vi "禹山浊度校准.vi"() -> ()   [LabVIEW 2016, in "斯坦道多参数.lvlib"]
uses:
  <vilib>/Utility/miscctls.llb/LVPointTypeDef.ctl
  <vilib>/Analysis/NI_AALBase.lvlib
  <vilib>/Analysis/NI_AALPro.lvlib
panel:
  out "滤波设定":dbl
  out "通讯状态":string
  out "第二点校准值":dbl
  out "第一点校准值":dbl
  out "最小值":sgl format="%.2g"
  out "最大值":sgl format="%.2g"
  in  "校准停止":bool
  in  "校准模式":u16(ring) items=["两点校准", "单点校准"]
  in  "标液2":dbl
  in  "标液1":dbl
  out "波形图表":sgl(graph) caption="历史曲线"
  out "温度测量值":dbl caption="温度" format="%#.2f"
  out "变异系数":dbl format="%.6g"
  out "standard deviation":dbl caption="标准差" format="%0.2f"
  out "mean":dbl caption="均值" format="%0.2f"
  out "提示":string
  in  "校准启动":bool
  out "测试值":dbl format="%#.2f"
  out "电极斜率":dbl format="%#.6f"
  out "电极零点":dbl format="%#.6f"
  # "浊度电极设定"
  # "℃"
  # "NTU"
  # "请选择校准模式:"
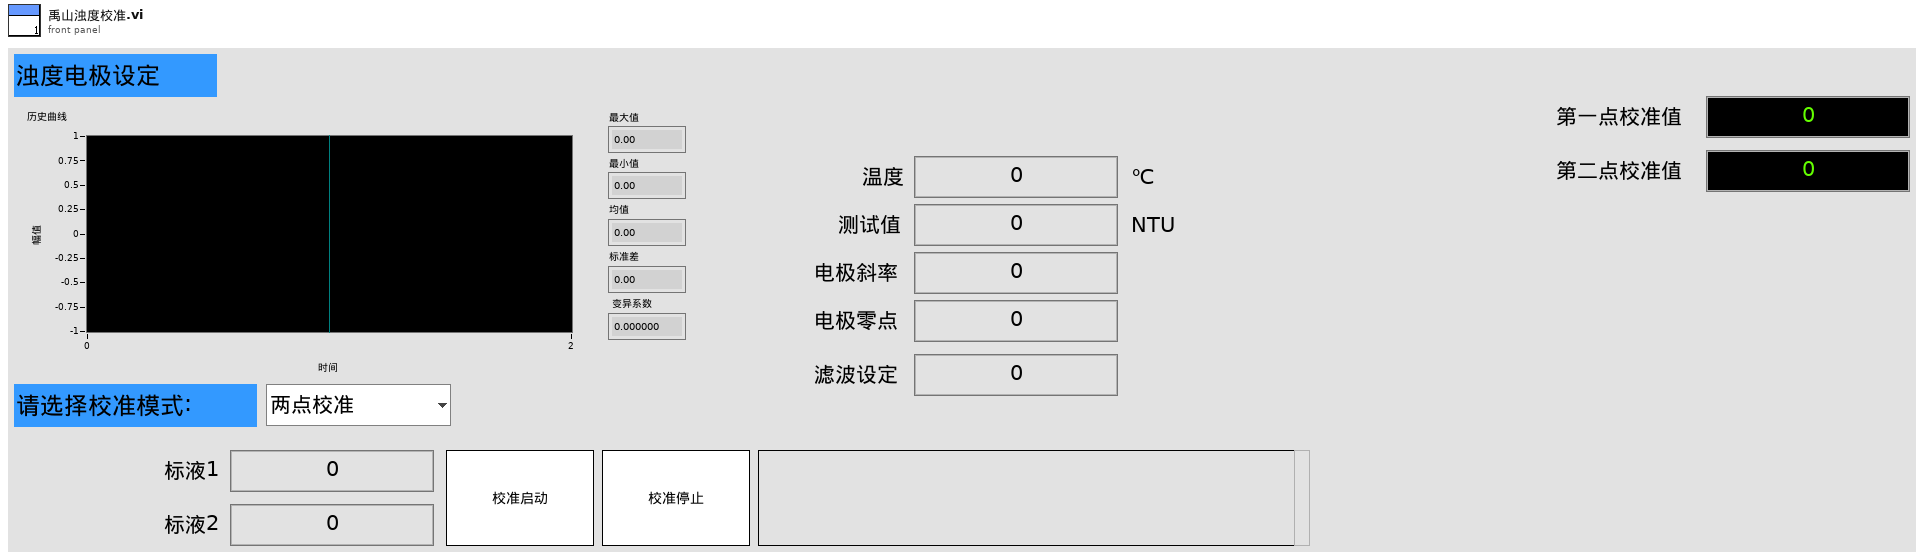
[diagram p1: front panel]
types:
  T1 = typedef "斯坦道多参数.lvlib/通知队列类型.ctl" = enum16{"pH", "DO", "DO2", "Cond", "Turb", "ORP", "叶绿素a", "藻密度", "COD"}
  T2 = typedef "LVPointTypeDef.ctl" = cluster{"Horizontal":i16, "Vertical":i16}
  T3 = cluster{"pH":u32, "DO":u32, "Cond":u32, "Turb":u32, "叶绿素a":u32, "藻密度":u32, "ORP":u32, "COD":u32}
  T4 = enum8{"Enabled", "Disabled", "Disabled and Grayed Out"}
  T5 = cluster{"ph":bool, "DO":bool, "Cond":bool, "Turb":bool, "叶绿素a":bool, "藻密度":bool, "ORP":bool, "COD":bool, "DO2":bool}
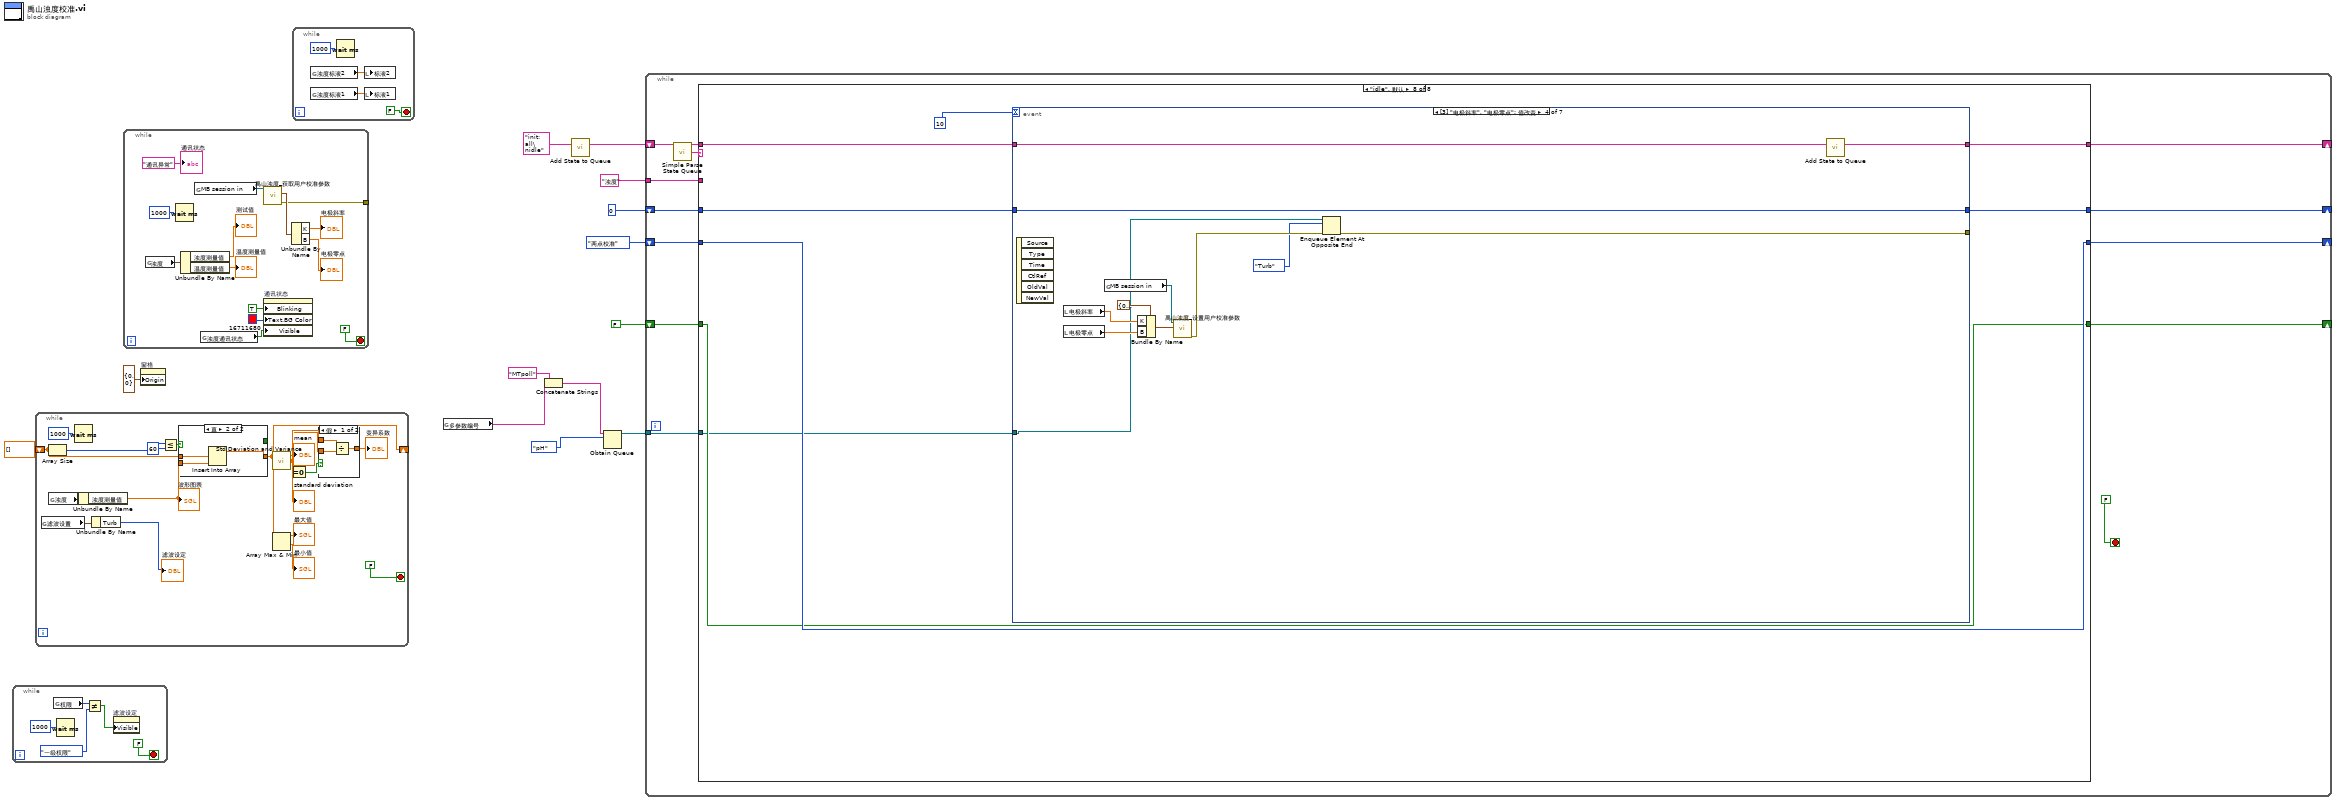
[diagram p0: block diagram]
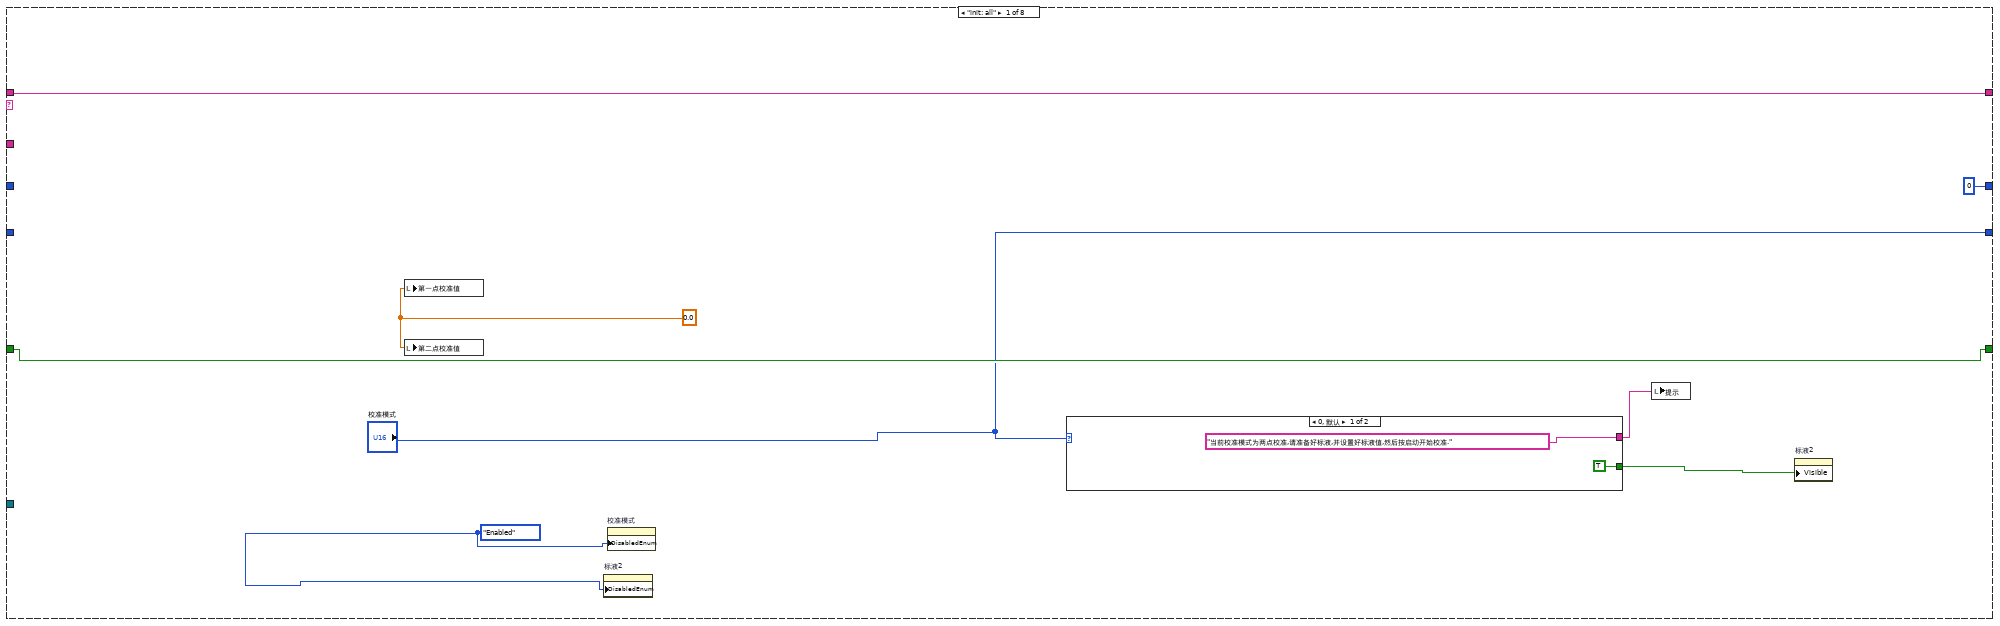
[diagram p2: hidden frame]
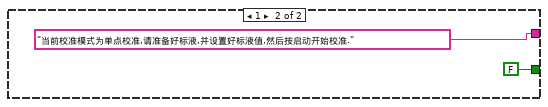
[diagram p3: hidden frame]
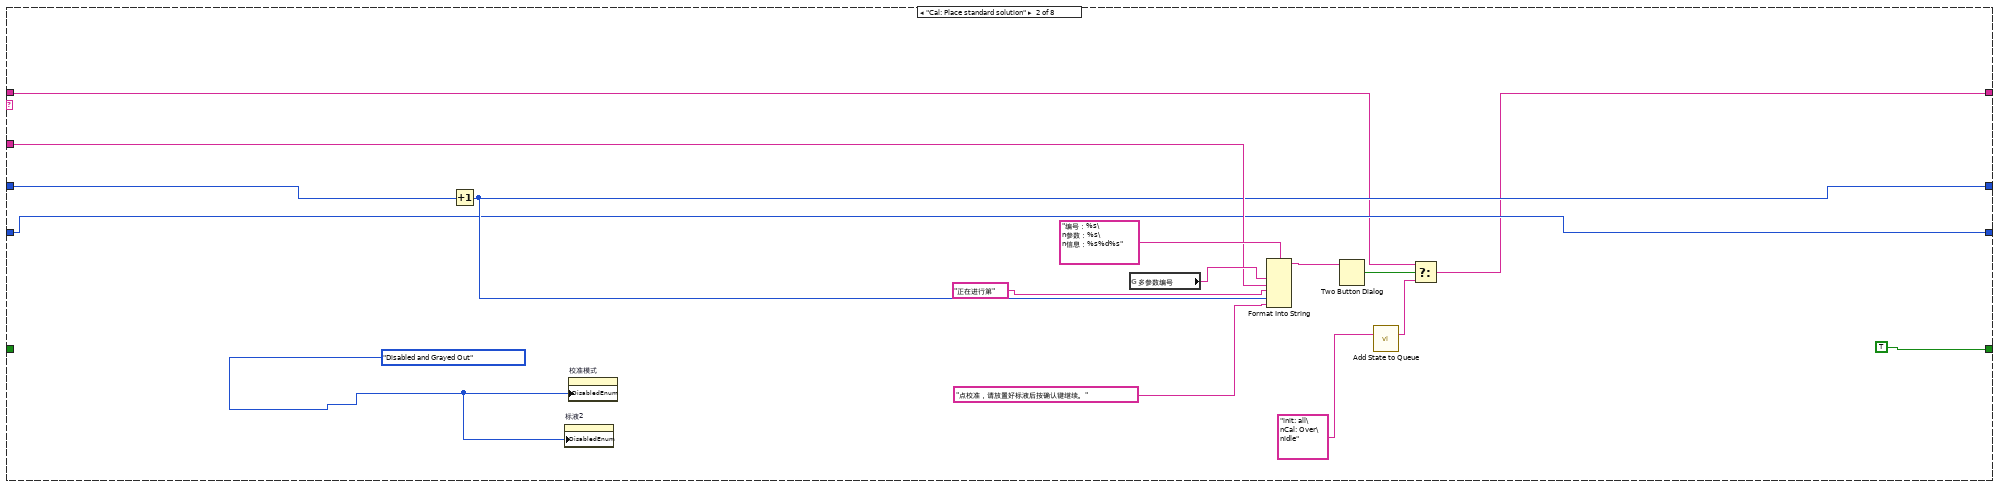
[diagram p4: hidden frame]
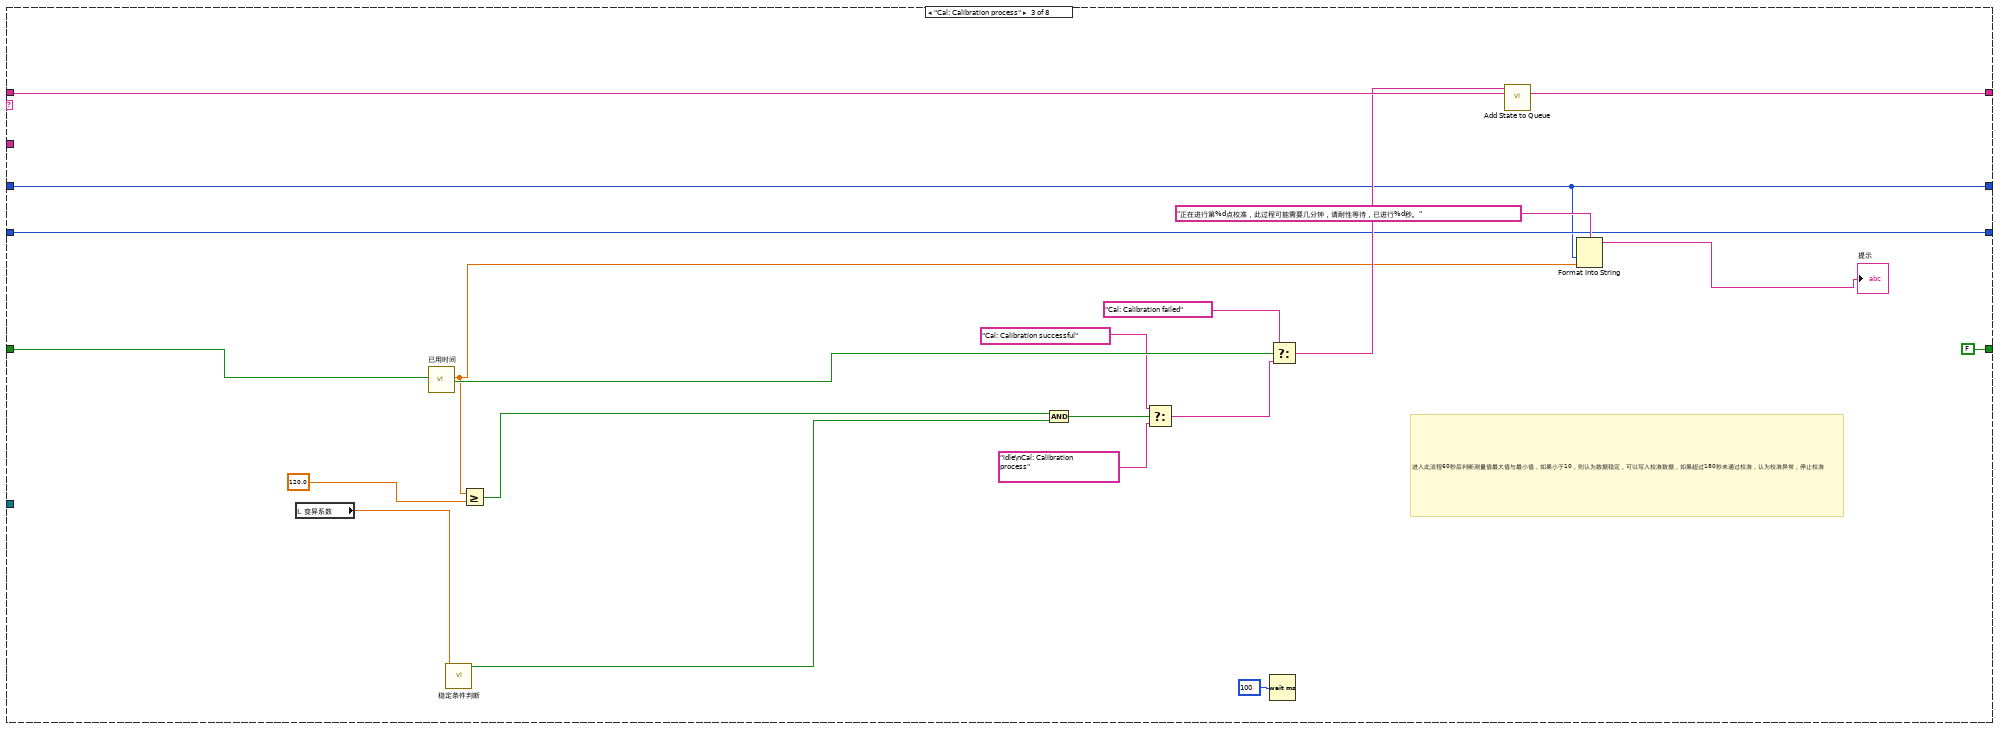
[diagram p5: hidden frame]
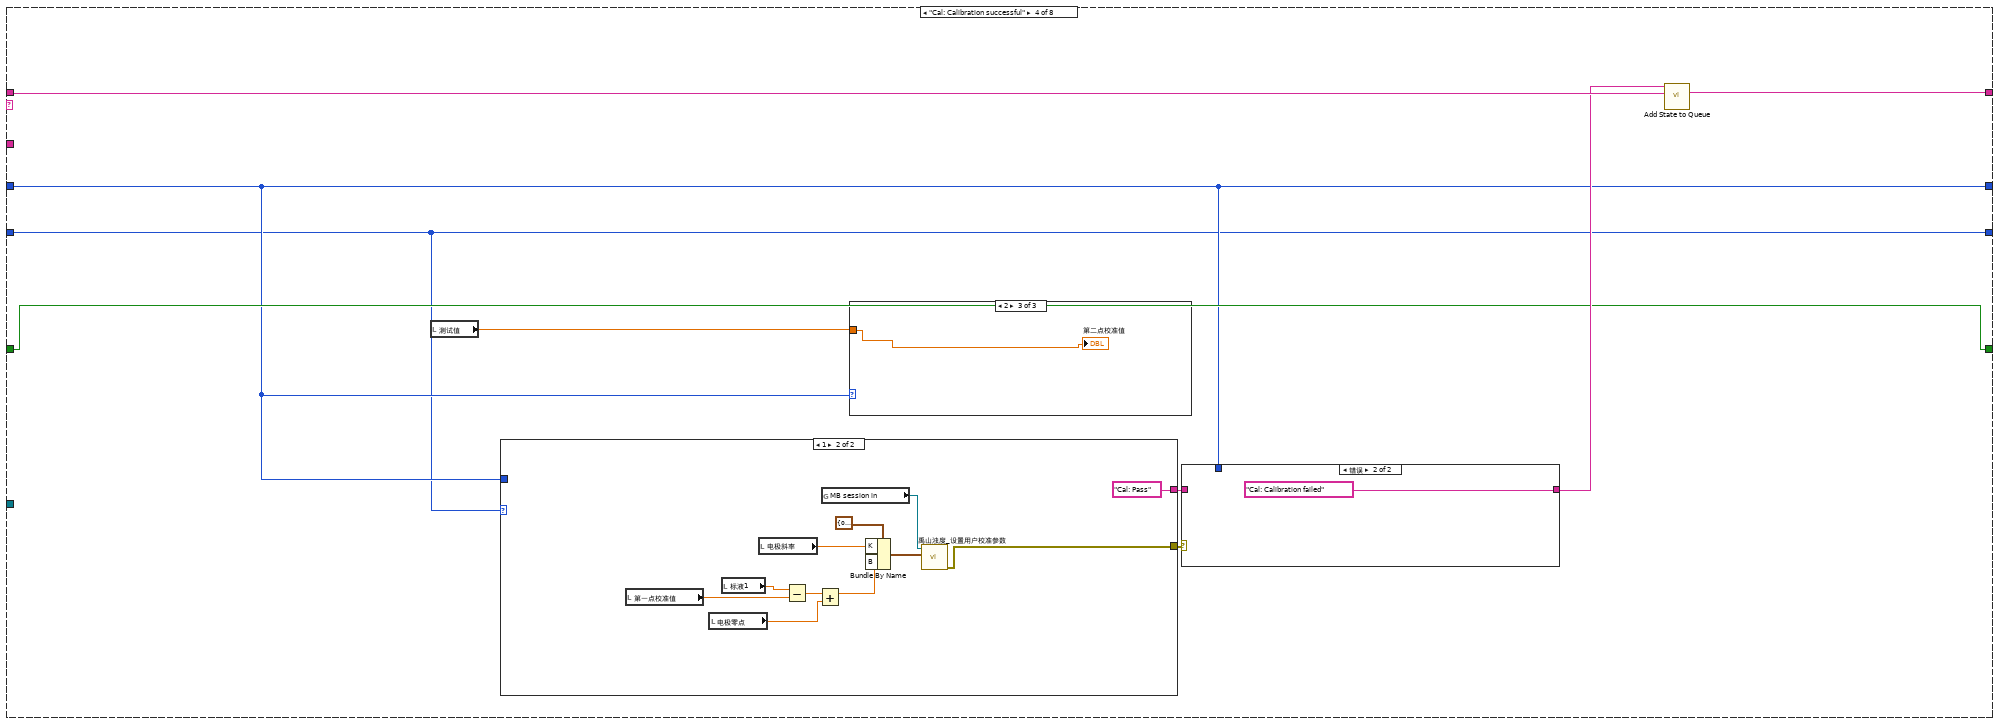
[diagram p6: hidden frame]
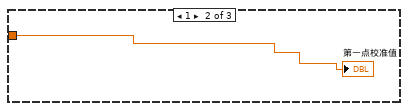
[diagram p8: hidden frame]
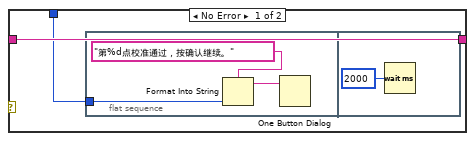
[diagram p9: hidden frame]
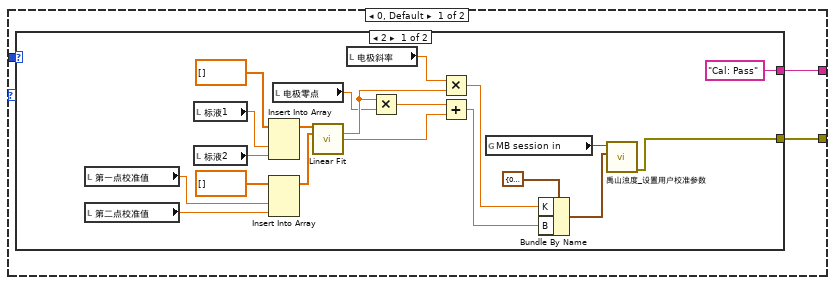
[diagram p10: hidden frame]
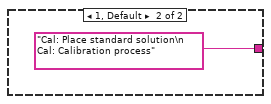
[diagram p11: hidden frame]
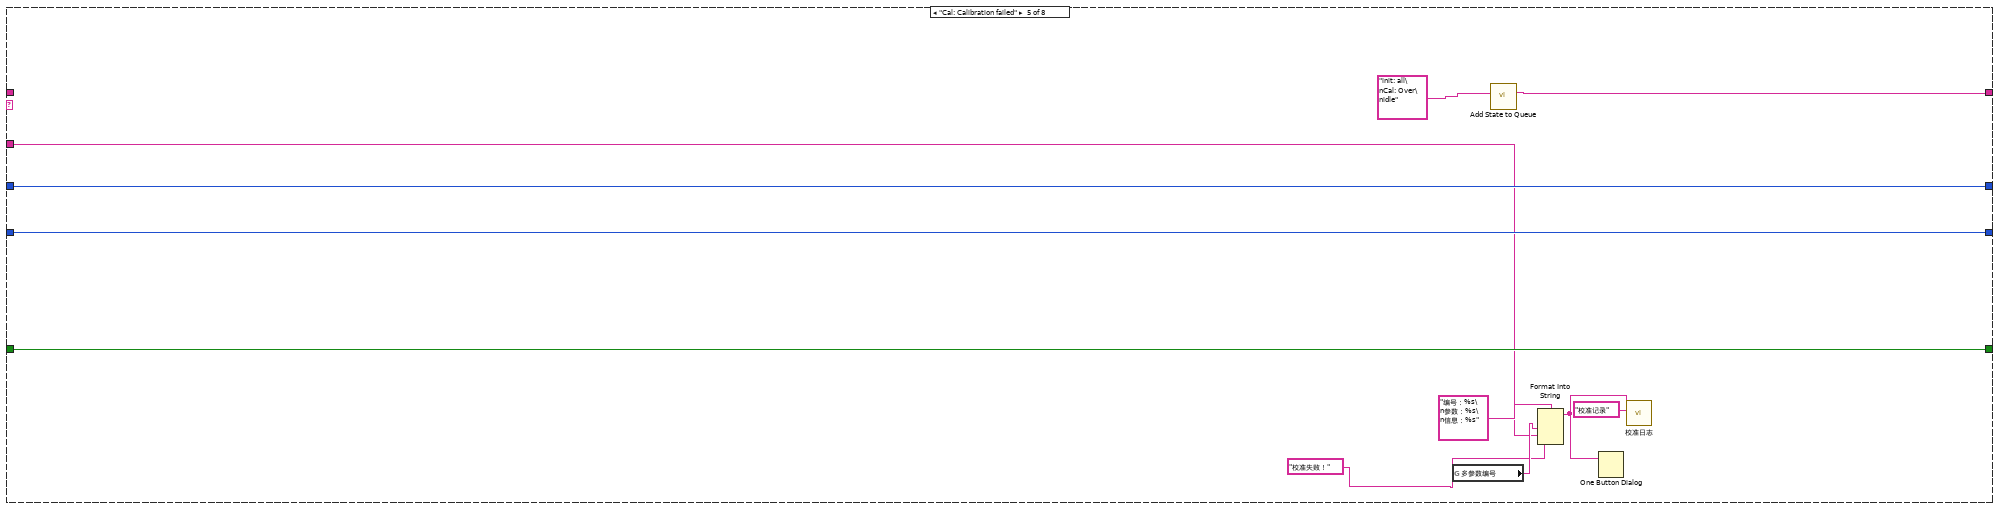
[diagram p12: hidden frame]
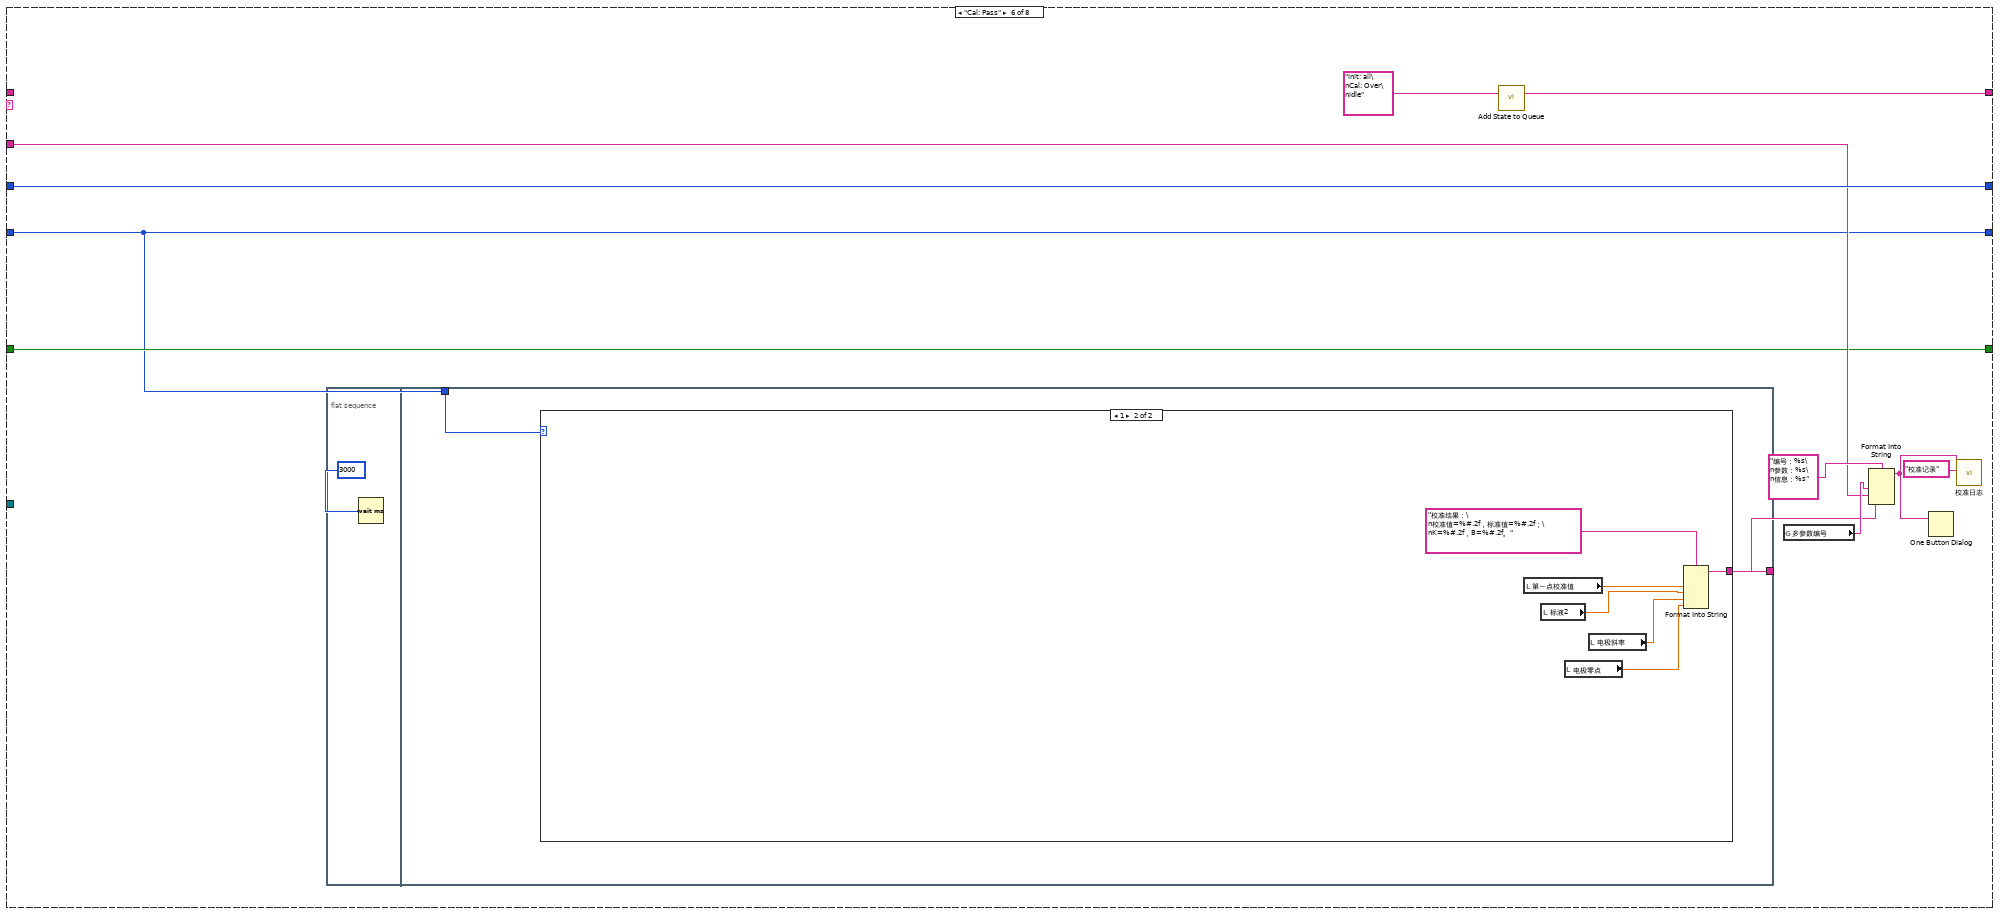
[diagram p13: hidden frame]
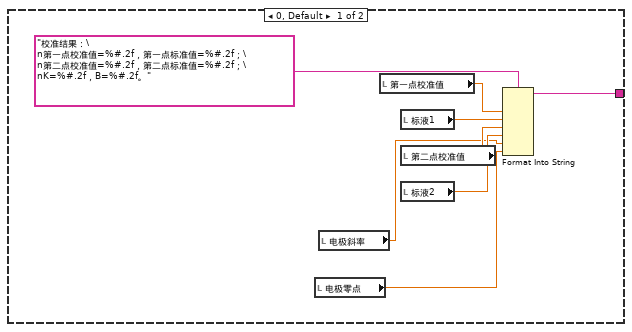
[diagram p14: hidden frame]
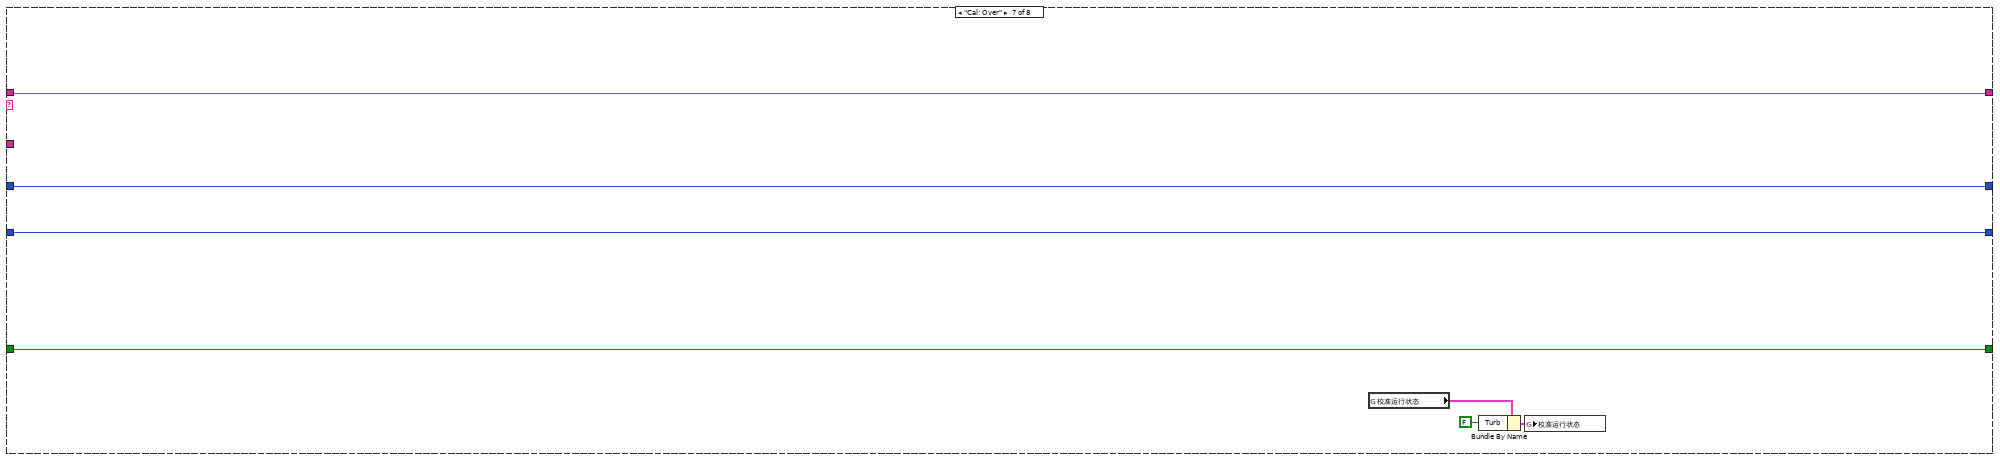
[diagram p15: hidden frame]
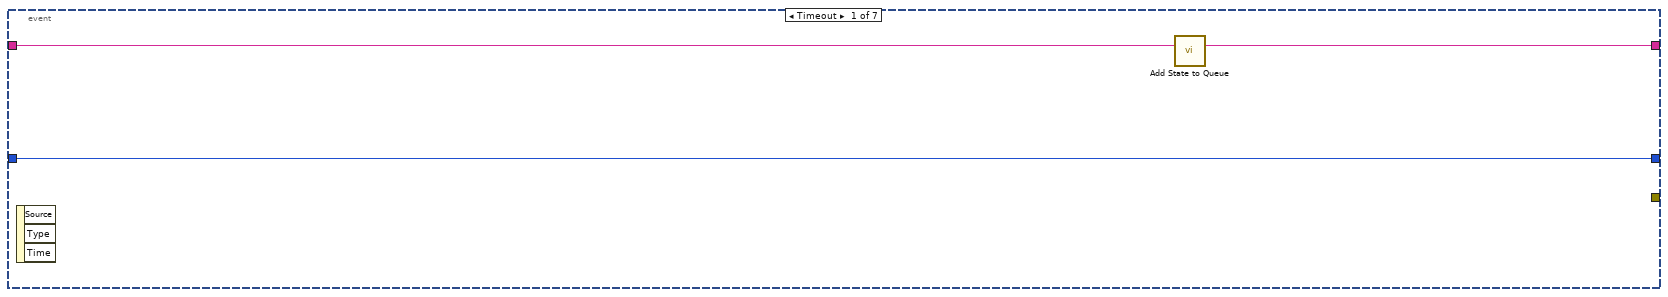
[diagram p16: hidden frame]
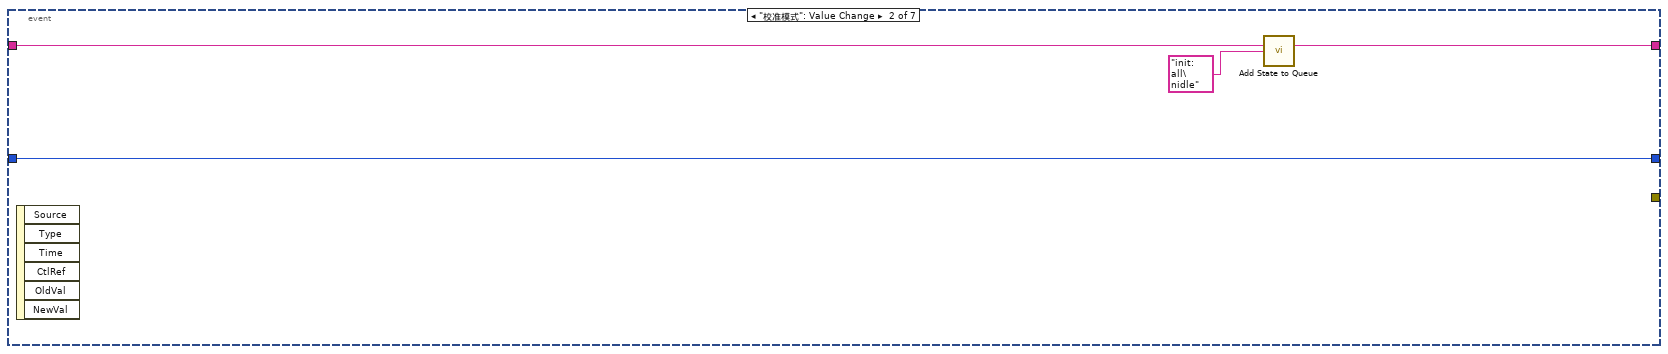
[diagram p17: hidden frame]
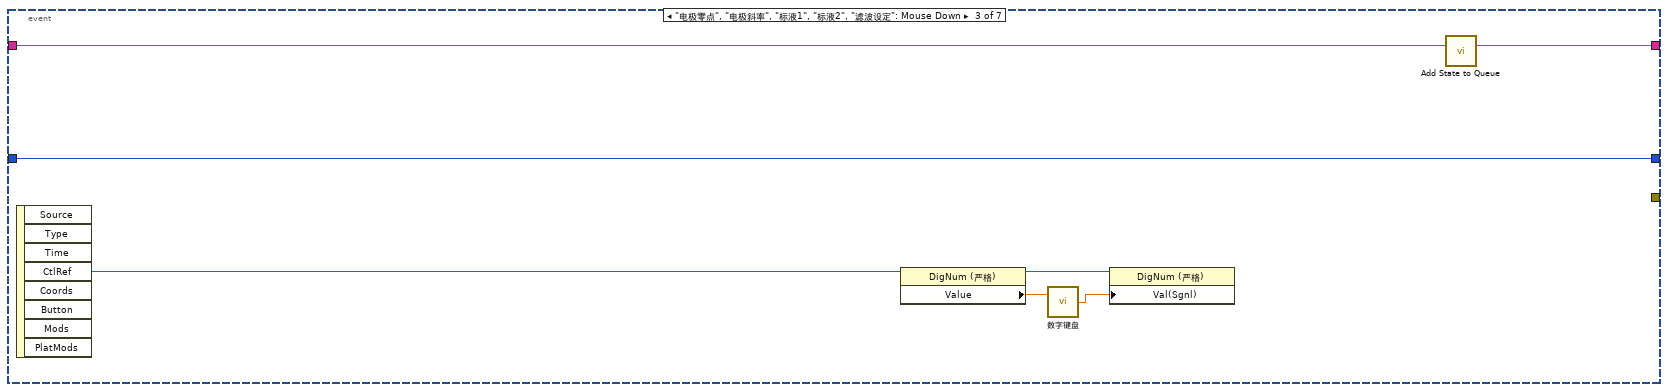
[diagram p18: hidden frame]
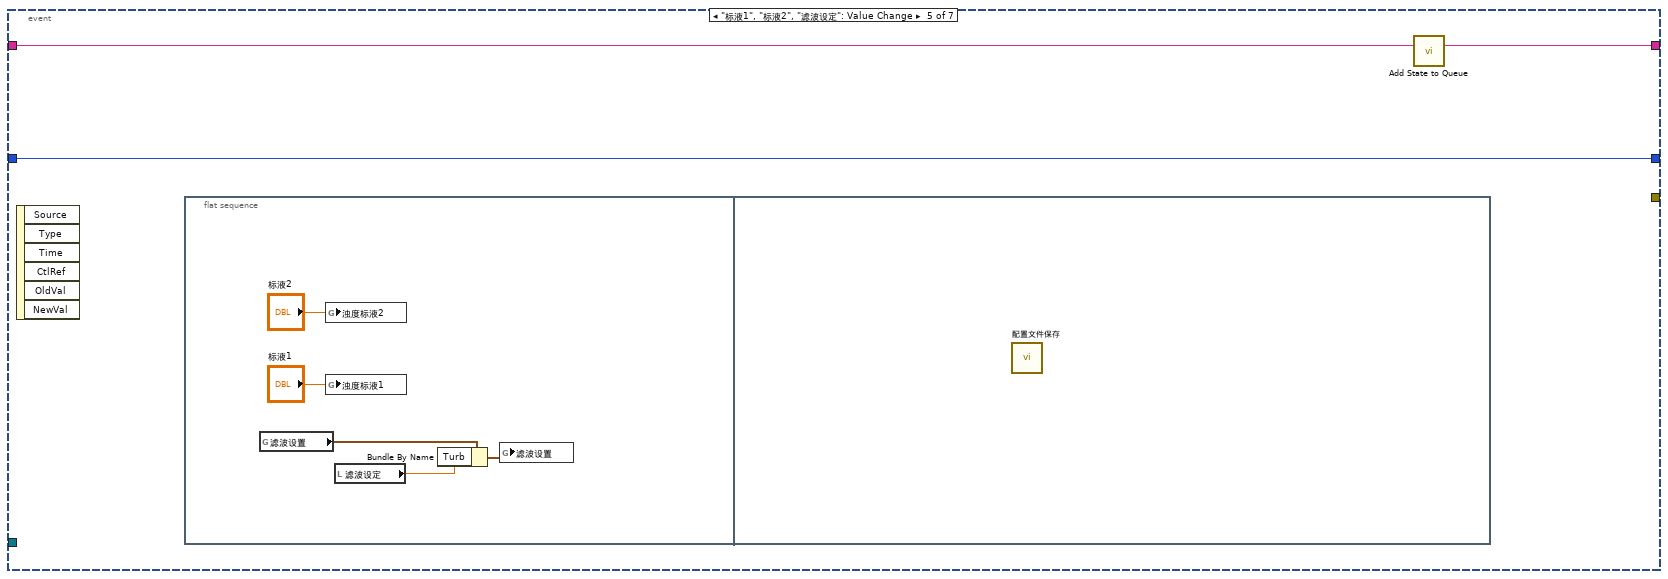
[diagram p19: hidden frame]
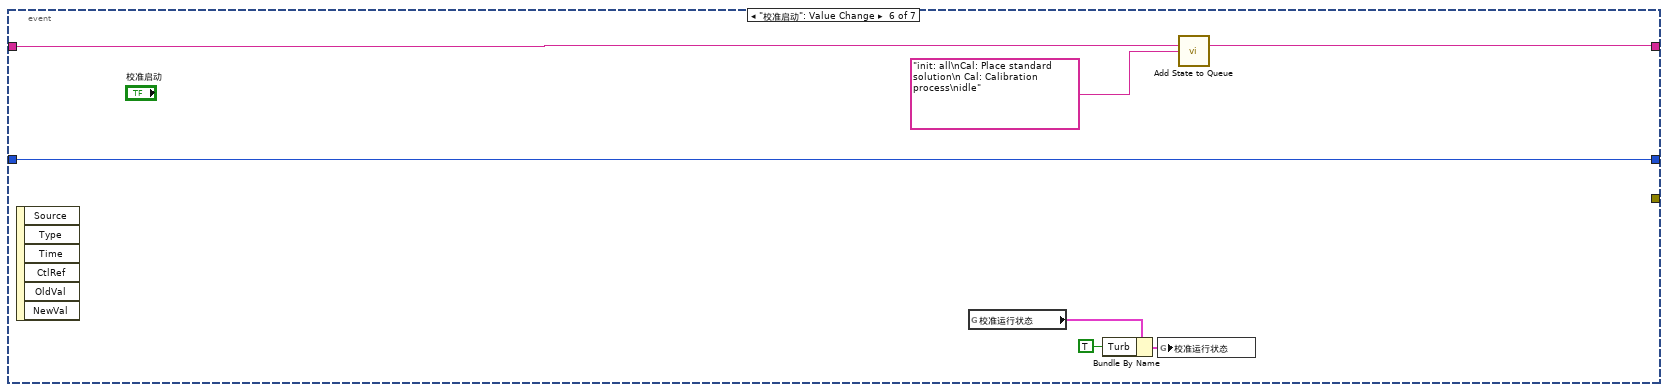
[diagram p20: hidden frame]
diagram:
  n1 = while {
    stop <- FALSE stop-if-true
    n2 = global read "多参数全局变量.vi" "权限"() -> (w17:enum16{"一级权限", "二级权限", "三级权限", "超级权限"})
    n3 = Wait (ms)(milliseconds to wait=u32 1000 ("等待时间（毫秒）")) -> ()  [unwired: 1 out]
    n4 = Not Equal?(x=w17, y=enum16{"一级权限", "二级权限", "三级权限"}."一级权限") -> (x != y?=w14:bool)
    n5 = property on="滤波设定" class="DigNum (严格)"("Visible"=w14) -> ()  [unwired: 2 in, 2 out]
  }
  n6 = while {
    shift-right: [w24] -> _
    shift-left: sgl[] [] -> [w31]
    stop <- FALSE stop-if-true
    n7 = global read "断电保存变量.vi" "滤波设置"() -> (w20:T3)
    n8 = Array Size(array=w31) -> (size(s)=w33:i32)
    n9 = global read "禹山过程全局变量.vi" "浊度"() -> (w25:cluster{"温度测量值":sgl, "浊度测量值":sgl})
    n10 = Wait (ms)(milliseconds to wait=u32 1000 ("等待时间（毫秒）")) -> ()  [unwired: 1 out]
    n11 = Unbundle By Name(w25) -> ("浊度测量值"=w21:sgl)
    "波形图表" <- w21
    n12 = Unbundle By Name(w20) -> ("Turb"=→"滤波设定":u32)
    n13 = Less Or Equal?(x=w33, y=60) -> (x <= y?=w32:bool)
    n14 = case shown="真" w32 {
      tunnel: w31 -> [w44 w47]
      tunnel: w21 -> [w42 w46]
      tunnel: [w40 w45] -> w24
      tunnel: [TRUE _] -> _
      frame False {
        n15 = Replace Array Subset(array=w44, new element=w42) -> (w43:sgl[])  [unwired: 1 in]
        n16 = Rotate 1D Array(1:w43, 2:-1 ("n")) -> (0:w40:sgl[])
      }
      frame True {
        n17 = Insert Into Array(array=w47, new element=w46) -> (w45:sgl[])  [unwired: 1 in]
      }
    }
    n18 = call <vilib>:"Std Deviation and Variance.vi"("X"=w24) -> ("mean"=w26:dbl, "standard deviation"=w27:dbl)  [unwired: 1 in, 1 out]
    "standard deviation" <- w27
    "mean" <- w26
    n19 = Array Max & Min(array=w24) -> (max value=→"最大值":sgl, min value=→"最小值":sgl)  [unwired: 2 out]
    n20 = Equal To 0?(x=w26) -> (x = 0?=w30:bool)
    n21 = case shown="假" w30 {
      tunnel: w27 -> [w38 _]
      tunnel: [w37 _] -> w29
      tunnel: w26 -> [w36 _]
      frame False {
        n22 = Divide(x=w38, y=w36) -> (x/y=w37:dbl)
      }
      frame True {
      }
    }
    "变异系数" <- w29
  }
  n23 = while {
    tunnel: [w56] -> _
    stop <- FALSE stop-if-true
    n24 = global read "禹山过程全局变量.vi" "浊度"() -> (w53:cluster{"温度测量值":sgl, "浊度测量值":sgl})
    n25 = Wait (ms)(milliseconds to wait=u32 1000 ("等待时间（毫秒）")) -> ()  [unwired: 1 out]
    n26 = Unbundle By Name(w53) -> ("浊度测量值"=→"测试值":sgl, "温度测量值"=→"温度测量值":sgl)
    n27 = global read "多参数全局变量.vi" "MB session in"() -> (w52:refnum<class "MB_Master.lvclass">)
    n28 = global read "多参数全局变量.vi" "浊度通讯状态"() -> (w48:bool)
    n29 = call "禹山浊度_获取用户校准参数.vi"("MB session in"=w52) -> ("error out"=w56:errorcluster, "输出值"=w59:cluster{"K":sgl, "B":sgl})  [unwired: 8 in, 1 out]
    n30 = property on="通讯状态" class="Str"("Blinking"=TRUE ("闪烁"), "Text.BG Color"=u32 16711680, "Visible"=w48) -> ()  [unwired: 2 in, 2 out]
    n31 = Unbundle By Name(w59) -> ("K"=→"电极斜率":sgl, "B"=→"电极零点":sgl)
    "通讯状态" <- "通讯异常" ("当前串口")
  }
  n32 = property on="窗格" class="Pane"("Origin"=T2 {"Horizontal"=0, "Vertical"=0} ("原点")) -> ()  [unwired: 2 in, 2 out]
  n33 = while {
    stop <- FALSE stop-if-true
    n34 = global read "断电保存变量.vi" "浊度标液2"() -> (w62:dbl)
    n35 = global read "断电保存变量.vi" "浊度标液1"() -> (w63:dbl)
    n36 = Wait (ms)(milliseconds to wait=u32 1000 ("等待时间（毫秒）")) -> ()  [unwired: 1 out]
    n37 = local write "标液2"(w62) -> ()
    n38 = local write "标液1"(w63) -> ()
  }
  n39 = global read "多参数全局变量.vi" "多参数编号"() -> (w3:string)
  n40 = Concatenate Strings("MTpoll" ("名称（未命名）"), w3) -> (w4:string)
  n41 = call "Add State to Queue.vi"("State(s) In (\"\")"="init: all\nidle" ("State(s) In (\"\")")) -> ("States Out"=w10:string)  [unwired: 14 in]
  n42 = Obtain Queue(name (unnamed)=w4, element data type=通知队列类型."pH" ("枚举")) -> (queue out=w2:refnum<queue>)  [unwired: 3 in, 2 out]
  n43 = while {
    shift-right: [w74] -> _
    shift-left: w10 -> [w78]
    shift-right: [w71] -> _
    shift-left: 0 -> [w73]
    tunnel: "浊度" ("State(s) In (\"\")") -> [w72]
    shift-right: [w69] -> _
    shift-left: enum16{"两点校准", "单点校准"}."两点校准" ("校准模式") -> [w70]
    shift-right: [w67] -> _
    shift-left: FALSE -> [w68]
    tunnel: w2 -> [w66]
    stop <- FALSE stop-if-true
    n44 = call "Simple Parse State Queue.vi"("State Queue"=w78) -> ("Remain States"=w75:string, "Next State"=w76:string)  [unwired: 13 in]
    n45 = case shown="\"idle\", 默认" w76 {
      tunnel: w75 -> [w86 w94 w126 w134 _ _ w226 w234]
      tunnel: [w86 w93 w125 w133 w188 w193 w226 w233] -> w74
      tunnel: w73 -> [_ w102 w111 w129 w191 w202 w225 w231]
      tunnel: w72 -> [_ w103 _ _ w182 w198 _ _]
      tunnel: [0 w100 w111 w129 w191 w202 w225 w232] -> w71
      tunnel: w70 -> [_ w99 w112 w128 w190 w194 w224 w230]
      tunnel: ["校准模式" w99 w112 w128 w190 w194 w224 w230] -> w69
      tunnel: w68 -> [w83 _ w114 w130 w189 w197 w223 w228]
      tunnel: [w83 TRUE FALSE w130 w189 w197 w223 w228] -> w67
      tunnel: w66 -> [_ _ _ _ _ _ _ w227]
      frame "init: all" {
        w82 = T4."Enabled" ("禁用")
        w79 = 0.0 ("第一点校准值")
        n46 = local write "第一点校准值"(w79) -> ()
        n47 = local write "第二点校准值"(w79) -> ()
        n48 = property on="标液2" class="DigNum (严格)"("DisabledEnum"=w82) -> ()  [unwired: 2 in, 2 out]
        n49 = property on="校准模式" class="Ring (严格)"("DisabledEnum"=w82) -> ()  [unwired: 2 in, 2 out]
        n50 = case shown="0, 默认" "校准模式" {
          tunnel: ["当前校准模式为两点校准,请准备好标液,并设置好标液值,然后按启动开始校准." ("提示") "当前校准模式为单点校准,请准备好标液,并设置好标液值,然后按启动开始校准." ("提示")] -> w85
          tunnel: [TRUE ("可见") FALSE ("可见")] -> w80
          frame 0, Default {
          }
          frame 1 {
          }
        }
        n51 = local write "提示"(w85) -> ()
        n52 = property on="标液2" class="DigNum (严格)"("Visible"=w80) -> ()  [unwired: 2 in, 2 out]
      }
      frame "Cal: Place standard solution" {
        w92 = T4."Disabled and Grayed Out" ("禁用")
        n53 = Increment(x=w102) -> (x+1=w100:i32)
        n54 = property on="标液2" class="DigNum (严格)"("DisabledEnum"=w92) -> ()  [unwired: 2 in, 2 out]
        n55 = property on="校准模式" class="Ring (严格)"("DisabledEnum"=w92) -> ()  [unwired: 2 in, 2 out]
        n56 = global read "多参数全局变量.vi" "多参数编号"() -> (w105:string)
        n57 = Format Into String(format string="编号：%s\n参数：%s\n信息：%s%d%s" ("格式字符串"), w105, w103, "正在进行第" ("消息"), w100, "点校准，请放置好标液后按确认键继续。" ("消息")) -> (resulting string=w97:string)  [unwired: 2 in, 1 out]
        n58 = Two Button Dialog(message=w97) -> (T button?=w96:bool)  [unwired: 2 in]
        n59 = call "Add State to Queue.vi"("State(s) In (\"\")"="init: all\nCal: Over\nidle" ("State(s) In (\"\")")) -> ("States Out"=w95:string)  [unwired: 14 in]
        n60 = Select(t=w94, s=w96, f=w95) -> (s? t:f=w93:string)
      }
      frame "Cal: Calibration process" {
        # "进入此流程60秒后判断测量值最大值与最小值，如果小于10，则认为数据稳定，可以写入校准数据，如果超过180秒未通过校准，认为校准异常，停止校准"
        n61 = local read "变异系数"() -> (w108:dbl)
        n62 = call "已用时间"("Reset"=w114) -> ("Elapsed Time (s)"=w110:dbl, "Time has Elapsed"=w127:bool)  [unwired: 11 in, 6 out]
        n63 = call "稳定条件判断.vi"("变异系数"=w108) -> ("布尔"=w107:bool)  [unwired: 10 in]
        n64 = Greater Or Equal?(x=w110, y=120.0) -> (x >= y?=w122:bool)
        n65 = And(x=w122, y=w107) -> (x .and. y?=w119:bool)
        n66 = Select(t="Cal: Calibration successful" ("State(s) In (\"\")"), s=w119, f="idle\nCal: Calibration process" ("State(s) In (\"\")")) -> (s? t:f=w118:string)
        n67 = Wait (ms)(milliseconds to wait=u32 100 ("等待时间（毫秒）")) -> ()  [unwired: 1 out]
        n68 = Select(t="Cal: Calibration failed" ("State(s) In (\"\")"), s=w127, f=w118) -> (s? t:f=w117:string)
        n69 = call "Add State to Queue.vi"("State(s) In Front (\"\")"=w117, "State(s) In (\"\")"=w126) -> ("States Out"=w125:string)  [unwired: 13 in]
        n70 = Format Into String(format string="正在进行第%d点校准，此过程可能需要几分钟，请耐性等待，已进行%d秒。" ("格式字符串"), w111, w110) -> (resulting string=→"提示":string)  [unwired: 2 in, 1 out]
      }
      frame "Cal: Calibration successful" {
        n71 = local read "测试值"() -> (w131:dbl)
        n72 = case shown="1" w128 {
          tunnel: [w148 w170] -> w136
          tunnel: [w147 "Cal: Pass" ("State(s) In (\"\")")] -> w135
          tunnel: w129 -> [w146 _]
          frame 0, Default {
            n73 = case shown="2" w146 {
              tunnel: [w149 _] -> w148
              tunnel: ["Cal: Pass" ("State(s) In (\"\")") "Cal: Place standard solution\n Cal: Calibration process" ("State(s) In (\"\")")] -> w147
              frame 2 {
                n74 = local read "第一点校准值"() -> (w166:dbl)
                n75 = local read "第二点校准值"() -> (w165:dbl)
                n76 = local read "标液1"() -> (w163:dbl)
                n77 = local read "标液2"() -> (w162:dbl)
                n78 = Insert Into Array(array=dbl[] [] ("Weight"), new element #1=w163, new element #2=w162) -> (w161:dbl[])  [unwired: 1 in]
                n79 = Insert Into Array(array=dbl[] [] ("Weight"), new element #1=w166, new element #2=w165) -> (w160:dbl[])  [unwired: 1 in]
                n80 = local read "电极零点"() -> (w153:dbl)
                n81 = call <vilib>:"Linear Fit.vi"("Y"=w161, "X"=w160) -> ("slope"=w154:dbl, "intercept"=w151:dbl)  [unwired: 9 in, 3 out]
                n82 = local read "电极斜率"() -> (w156:dbl)
                n83 = Multiply(x=w154, y=w153) -> (x*y=w152:dbl)
                n84 = Multiply(x=w156, y=w154) -> (x*y=w155:dbl)
                n85 = Add(x=w152, y=w151) -> (x+y=w150:dbl)
                n86 = global read "多参数全局变量.vi" "MB session in"() -> (w159:refnum<class "MB_Master.lvclass">)
                n87 = Bundle By Name(cluster=cluster{"K":sgl, "B":sgl} {"K"=0.0, "B"=0.0} ("用户校准参数"), "K"=w155, "B"=w150) -> (w158:cluster{"K":sgl, "B":sgl})
                n88 = call "禹山浊度_设置用户校准参数.vi"("用户校准参数"=w158, "MB session in"=w159) -> ("error out"=w149:errorcluster)  [unwired: 8 in, 1 out]
              }
              frame 1, Default {
              }
            }
          }
          frame 1 {
            n89 = local read "第一点校准值"() -> (w175:dbl)
            n90 = local read "电极零点"() -> (w179:dbl)
            n91 = local read "标液1"() -> (w176:dbl)
            n92 = local read "电极斜率"() -> (w174:dbl)
            n93 = Subtract(x=w176, y=w175) -> (x-y=w177:dbl)
            n94 = Add(x=w177, y=w179) -> (x+y=w178:dbl)
            n95 = global read "多参数全局变量.vi" "MB session in"() -> (w171:refnum<class "MB_Master.lvclass">)
            n96 = Bundle By Name(cluster=cluster{"K":sgl, "B":sgl} {"K"=0.0, "B"=0.0} ("用户校准参数"), "K"=w174, "B"=w178) -> (w172:cluster{"K":sgl, "B":sgl})
            n97 = call "禹山浊度_设置用户校准参数.vi"("用户校准参数"=w172, "MB session in"=w171) -> ("error out"=w170:errorcluster)  [unwired: 8 in, 1 out]
          }
        }
        n98 = case shown="2" w129 {
          tunnel: w131 -> [_ w137 w138]
          frame 0, Default {
          }
          frame 1 {
            "第一点校准值" <- w137
          }
          frame 2 {
            "第二点校准值" <- w138
          }
        }
        n99 = case shown="错误" w136 {
          tunnel: w135 -> [w140 _]
          tunnel: [w140 "Cal: Calibration failed" ("State(s) In (\"\")")] -> w132
          tunnel: w129 -> [w139 _]
          frame No Error {
            n100 = flat-sequence {
              tunnel: w139 -> [w141]
              frame #0 {
                n101 = Format Into String(format string="第%d点校准通过，按确认继续。" ("格式字符串"), w141) -> (resulting string=w143:string)  [unwired: 2 in, 1 out]
                n102 = One Button Dialog(message=w143) -> ()  [unwired: 1 in, 1 out]
              }
              frame #1 {
                n103 = Wait (ms)(milliseconds to wait=u32 2000 ("等待时间（毫秒）")) -> ()  [unwired: 1 out]
              }
            }
          }
          frame Error {
          }
        }
        n104 = call "Add State to Queue.vi"("State(s) In Front (\"\")"=w132, "State(s) In (\"\")"=w134) -> ("States Out"=w133:string)  [unwired: 13 in]
      }
      frame "Cal: Calibration failed" {
        n105 = global read "多参数全局变量.vi" "多参数编号"() -> (w185:string)
        n106 = call "Add State to Queue.vi"("State(s) In (\"\")"="init: all\nCal: Over\nidle" ("State(s) In (\"\")")) -> ("States Out"=w188:string)  [unwired: 14 in]
        n107 = Format Into String(format string="编号：%s\n参数：%s\n信息：%s" ("格式字符串"), w185, w182, "校准失败！" ("消息")) -> (resulting string=w184:string)  [unwired: 2 in, 1 out]
        n108 = One Button Dialog(message=w184) -> ()  [unwired: 1 in, 1 out]
        n109 = call "校准日志.vi"("table"="校准记录", "日志信息"=w184) -> ()  [unwired: 9 in, 1 out]
      }
      frame "Cal: Pass" {
        n110 = flat-sequence {
          tunnel: [w205] -> w195
          tunnel: w194 -> [w204]
          frame #0 {
            n111 = Wait (ms)(milliseconds to wait=u32 3000 ("等待时间（毫秒）")) -> ()  [unwired: 1 out]
          }
          frame #1 {
            n112 = case shown="1" w204 {
              tunnel: [w213 w219] -> w205
              frame 0, Default {
                n113 = local read "电极零点"() -> (w206:dbl)
                n114 = local read "电极斜率"() -> (w207:dbl)
                n115 = local read "第一点校准值"() -> (w211:dbl)
                n116 = local read "标液1"() -> (w212:dbl)
                n117 = local read "第二点校准值"() -> (w209:dbl)
                n118 = local read "标液2"() -> (w208:dbl)
                n119 = Format Into String(format string="校准结果：\n第一点校准值=%#.2f，第一点标准值=%#.2f；\n第二点校准值=%#.2f，第二点标准值=%#.2f；\nK=%#.2f，B=%#.2f。" ("提示"), w211, w212, w209, w208, w207, w206) -> (resulting string=w213:string)  [unwired: 2 in, 1 out]
              }
              frame 1 {
                n120 = local read "第一点校准值"() -> (w218:dbl)
                n121 = local read "标液2"() -> (w216:dbl)
                n122 = local read "电极零点"() -> (w214:dbl)
                n123 = local read "电极斜率"() -> (w215:dbl)
                n124 = Format Into String(format string="校准结果：\n校准值=%#.2f，标准值=%#.2f；\nK=%#.2f，B=%#.2f。" ("提示"), w218, w216, w215, w214) -> (resulting string=w219:string)  [unwired: 2 in, 1 out]
              }
            }
          }
        }
        n125 = call "Add State to Queue.vi"("State(s) In (\"\")"="init: all\nCal: Over\nidle" ("State(s) In (\"\")")) -> ("States Out"=w193:string)  [unwired: 14 in]
        n126 = global read "多参数全局变量.vi" "多参数编号"() -> (w199:string)
        n127 = Format Into String(format string="编号：%s\n参数：%s\n信息：%s" ("格式字符串"), w199, w198, w195) -> (resulting string=w196:string)  [unwired: 2 in, 1 out]
        n128 = One Button Dialog(message=w196) -> ()  [unwired: 1 in, 1 out]
        n129 = call "校准日志.vi"("table"="校准记录", "日志信息"=w196) -> ()  [unwired: 9 in, 1 out]
      }
      frame "Cal: Over" {
        n130 = global read "多参数全局变量.vi" "校准运行状态"() -> (w221:T5)
        n131 = Bundle By Name(cluster=w221, "Turb"=FALSE) -> (w222:T5)
        n132 = global write "多参数全局变量.vi" "校准运行状态"(w222) -> ()
      }
      frame "idle", Default {
        n133 = event shown="[3] \"电极斜率\", \"电极零点\": 值改变" {
          selector: _ -> [_ _ _ _ _ _ _]
          dyn-events: _ -> [_ _ _ _ _ _ _]
          timeout: 10 -> [_ _ _ _ _ _ _]
          tunnel: [_ _ _ w251 _ _ _] -> _
          tunnel: w234 -> [w237 w241 w246 w252 w261 w275 _]
          tunnel: [w236 w240 w247 w259 w262 w274 w277] -> w233
          tunnel: [w235 w238 w248 w260 w263 w272 w278] -> w232
          tunnel: w231 -> [w235 w238 w248 w260 w263 w272 w278]
          tunnel: w227 -> [_ _ _ w250 _ _ _]
          event Timeout {
            n134 = event-data() -> ()  [unwired: 1 in, 3 out]
            n135 = call "Add State to Queue.vi"("State(s) In (\"\")"=w237) -> ("States Out"=w236:string)  [unwired: 14 in]
          }
          event "校准模式": Value Change {
            n136 = event-data() -> ()  [unwired: 1 in, 6 out]
            n137 = call "Add State to Queue.vi"("State(s) In (\"\")"=w241, "State(s) At Back (\"\")"="init: all\nidle" ("State(s) In (\"\")")) -> ("States Out"=w240:string)  [unwired: 13 in]
          }
          event "电极零点", "电极斜率", "标液1", "标液2", "滤波设定": Mouse Down {
            n138 = event-data() -> ("CtlRef"=w245:refnum<vi>)  [unwired: 1 in, 7 out]
            n139 = property class="DigNum (严格)"(reference=w245) -> (reference out=w242:refnum<vi>, "Value"=w243:dbl)  [unwired: 1 in, 1 out]
            n140 = call "数字键盘.vi"("OldNumber"=w243) -> ("NewNumber"=w244:dbl)  [unwired: 1 in]
            n141 = property class="DigNum (严格)"(reference=w242, "Val(Sgnl)"=w244) -> ()  [unwired: 1 in, 2 out]
            n142 = call "Add State to Queue.vi"("State(s) In (\"\")"=w246) -> ("States Out"=w247:string)  [unwired: 14 in]
          }
          event "电极斜率", "电极零点": Value Change {
            n143 = event-data() -> ()  [unwired: 1 in, 6 out]
            n144 = local read "电极斜率"() -> (w256:dbl)
            n145 = local read "电极零点"() -> (w257:dbl)
            n146 = global read "多参数全局变量.vi" "MB session in"() -> (w258:refnum<class "MB_Master.lvclass">)
            n147 = Bundle By Name(cluster=cluster{"K":sgl, "B":sgl} {"K"=0.0, "B"=0.0} ("用户校准参数"), "K"=w256, "B"=w257) -> (w255:cluster{"K":sgl, "B":sgl})
            n148 = call "禹山浊度_设置用户校准参数.vi"("用户校准参数"=w255, "MB session in"=w258) -> ("error out"=w253:errorcluster)  [unwired: 8 in, 1 out]
            n149 = Enqueue Element At Opposite End(queue=w250, element=通知队列类型."Turb" ("枚举"), error in (no error)=w253) -> (error out=w251:errorcluster)  [unwired: 1 in, 2 out]
            n150 = call "Add State to Queue.vi"("State(s) In (\"\")"=w252) -> ("States Out"=w259:string)  [unwired: 14 in]
          }
          event "标液1", "标液2", "滤波设定": Value Change {
            n151 = event-data() -> ()  [unwired: 1 in, 6 out]
            n152 = flat-sequence {
              frame #0 {
                n153 = global read "断电保存变量.vi" "滤波设置"() -> (w266:T3)
                n154 = global write "断电保存变量.vi" "浊度标液2"("标液2") -> ()
                n155 = global write "断电保存变量.vi" "浊度标液1"("标液1") -> ()
                n156 = local read "滤波设定"() -> (w264:dbl)
                n157 = Bundle By Name(cluster=w266, "Turb"=w264) -> (w265:T3)
                n158 = global write "断电保存变量.vi" "滤波设置"(w265) -> ()
              }
              frame #1 {
                n159 = call "配置文件保存.vi"() -> ()  [unwired: 12 in]
              }
            }
            n160 = call "Add State to Queue.vi"("State(s) In (\"\")"=w261) -> ("States Out"=w262:string)  [unwired: 14 in]
          }
          event "校准启动": Value Change {
            n161 = event-data() -> ()  [unwired: 1 in, 6 out]
            n162 = global read "多参数全局变量.vi" "校准运行状态"() -> (w270:T5)
            n163 = Bundle By Name(cluster=w270, "Turb"=TRUE) -> (w271:T5)
            n164 = global write "多参数全局变量.vi" "校准运行状态"(w271) -> ()
            n165 = call "Add State to Queue.vi"("State(s) In (\"\")"=w275, "State(s) At Back (\"\")"="init: all\nCal: Place standard solution\n Cal: Calibration process\nidle" ("State(s) In (\"\")")) -> ("States Out"=w274:string)  [unwired: 13 in]
          }
          event "校准停止": Value Change {
            n166 = event-data() -> ()  [unwired: 1 in, 6 out]
            n167 = call "Add State to Queue.vi"("State(s) In (\"\")"="init: all\nCal: Over\nidle" ("State(s) In (\"\")")) -> ("States Out"=w277:string)  [unwired: 14 in]
          }
        }
      }
    }
  }
